vi "GetTargetCandidates.vi"(9 "Minimum Area":dbl, 10 "HSL Range":T3={"Hue"={0.0, 6.122448979591837}, "Saturation"={0.0, 6.122448979591837}, "Luminance"={0.0, 6.122448979591837}} {"Luminance" scale=0.0..255.0; "Saturation" scale=0.0..255.0; "Hue" scale=0.0..255.0}, 11 "Image":T2) -> (1 "Thresholded Image":T2, 2 "Horizontal Targets":T1[](array[typedef]), 3 "Vertical Targetss":T1[](array[typedef]))   [LabVIEW 2013]
uses:
  <vilib>/vision/Image Controls.llb/IMAQ Image.ctl
  HSLRange.ctl
  Target Type.ctl
  <vilib>/vision/NI_Vision_Development_Module.lvlib
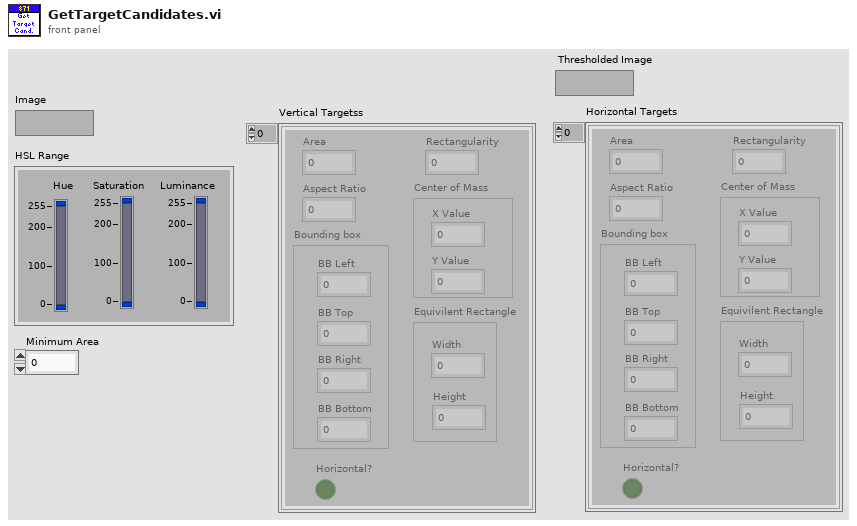
[diagram p1: front panel]
types:
  T1 = typedef "Target Type.ctl" = cluster{"Area":dbl, "Bounding box":cluster{"BB Left":dbl, "BB Top":dbl, "BB Right":dbl, "BB Bottom":dbl}, "Center of Mass":cluster{"X Value":dbl, "Y Value":dbl}, "Equivilent Rectangle":cluster{"Width":dbl, "Height":dbl}, "Aspect Ratio":dbl, "Rectangularity":dbl, "Horizontal?":bool}
  T2 = typedef "IMAQ Image.ctl" = refnum<image>
  T3 = typedef "HSLRange.ctl" = cluster{"Hue":cluster{dbl, dbl}, "Saturation":cluster{dbl, dbl}, "Luminance":cluster{dbl, dbl}}
  T4 = typedef "Particle Parameters" = i32
  T5 = typedef "Image Type" = u32
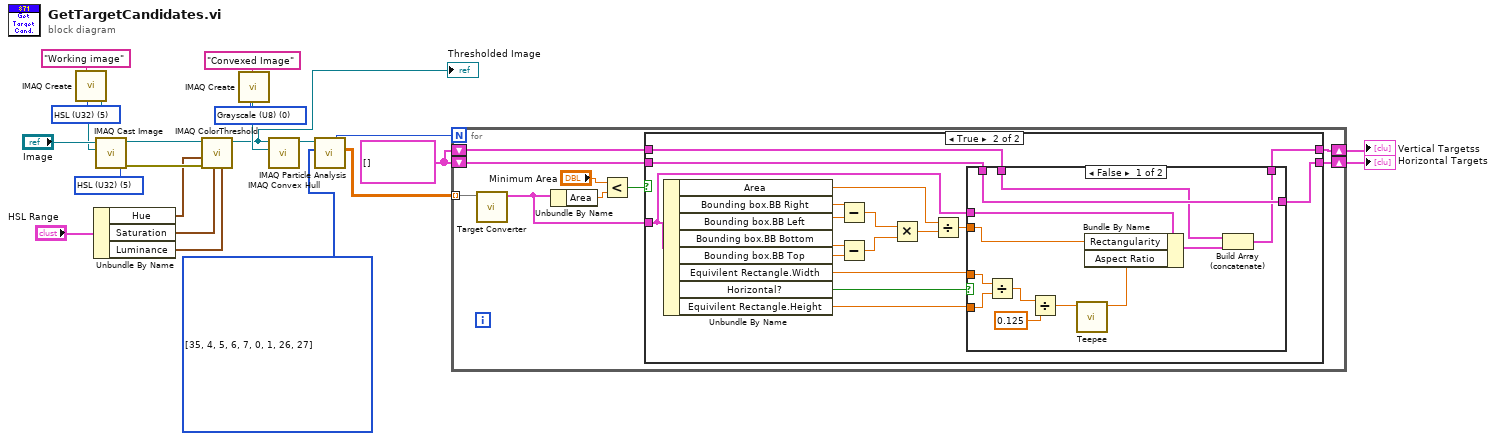
[diagram p0: block diagram]
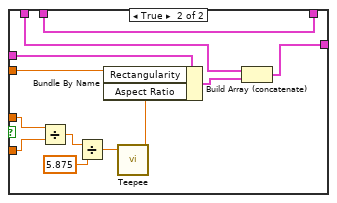
[diagram p3: hidden frame]
diagram:
  w4 = T4[] [35, 4, 5, 6, 7, 0, 1, 26, 27] items=["Center of Mass X", "Center of Mass Y", "First Pixel X", "First Pixel Y", "Bounding Rect Left", "Bounding Rect Top", "Bounding Rect Right", "Bounding Rect Bottom", "Max Feret Diameter Start X", "Max Feret Diameter Start Y", "Max Feret Diameter End X", "Max Feret Diameter End Y", "Max Horiz. Segment Length Left", "Max Horiz. Segment Length Right", "Max Horiz. Segment Length Row", "-", "Bounding Rect Width", "Bounding Rect Height", "Bounding Rect Diagonal", "Perimeter", "Convex Hull Perimeter", "Holes' Perimeter", "Max Feret Diameter", "Equivalent Ellipse Major Axis", "Equivalent Ellipse Minor Axis", "Equivalent Ellipse Minor Axis (Feret)", "Equivalent Rect Long Side", "Equivalent Rect Short Side", "Equivalent Rect Diagonal", "Equivalent Rect Short Side (Feret)", "Average Horiz. Segment Length", "Average Vert. Segment Length", "Hydraulic Radius", "Waddel Disk Diameter", "-", "Area", "Holes' Area", "Particle & Holes' Area", "Convex Hull Area", "Image Area", "-", "Number of Holes", "Number of Horiz. Segments", "Number of Vert. Segments", "-", "Orientation", "Max Feret Diameter Orientation", "-", "% Area/Image Area", "% Area/(Particle & Holes' Area)", "Ratio of Equivalent Ellipse Axes", "Ratio of Equivalent Rect Sides", "-", "Elongation Factor", "Compactness Factor", "Heywood Circularity Factor", "Type Factor", "-", "Sum X", "Sum Y", "Sum XX", "Sum XY", "Sum YY", "Sum XXX", "Sum XXY", "Sum XYY", "Sum YYY", "-", "Moment of Inertia XX", "Moment of Inertia XY", "Moment of Inertia YY", "Moment of Inertia XXX", "Moment of Inertia XXY", "Moment of Inertia XYY", "Moment of Inertia YYY", "Norm. Moment of Inertia XX", "Norm. Moment of Inertia XY", "Norm. Moment of Inertia YY", "Norm. Moment of Inertia XXX", "Norm. Moment of Inertia XXY", "Norm. Moment of Inertia XYY", "Norm. Moment of Inertia YYY", "Hu Moment 1", "Hu Moment 2", "Hu Moment 3", "Hu Moment 4", "Hu Moment 5", "Hu Moment 6", "Hu Moment 7"] ("Pixel Measurements")
  w3 = T1[] []
  w11 = T5 0 items=["Grayscale (U8)", "Grayscale (I16)", "Grayscale (SGL)", "Complex (CSG)", "RGB (U32)", "HSL (U32)", "RGB (U64)", "Grayscale (U16)"] ("Image Type")
  w18 = T5 5 items=["Grayscale (U8)", "Grayscale (I16)", "Grayscale (SGL)", "Complex (CSG)", "RGB (U32)", "HSL (U32)", "RGB (U64)", "Grayscale (U16)"] ("Image Type")
  w22 = T5 5 items=["Grayscale (U8)", "Grayscale (I16)", "Grayscale (SGL)", "Complex (CSG)", "RGB (U32)", "HSL (U32)", "RGB (U64)", "Grayscale (U16)"] ("Image Type")
  n1 = call "IMAQ Create"("Image Name"="Working image", "Image Type"=w18) -> ("New Image"=w16:T2)  [unwired: 3 in, 1 out]
  n2 = Unbundle By Name("HSL Range") -> ("Hue"=w14:cluster{dbl, dbl}, "Saturation"=w13:cluster{dbl, dbl}, "Luminance"=w12:cluster{dbl, dbl})
  n3 = call "IMAQ Cast Image"("Image Type"=w22, "Image Dst"=w16, "Image Src"="Image") -> ("error out"=w17:errorcluster, "Image Dst Out"=w20:T2)  [unwired: 7 in]
  n4 = call "IMAQ ColorThreshold"("Blue or Luma or Val or Inten Range"=w12, "Green or Sat Range"=w13, "error in (no error)"=w17, "Red or Hue Range"=w14, "Image Src"=w20) -> ("Image Dst Out"=w5:T2)  [unwired: 5 in, 1 out]
  "Thresholded Image" <- w5
  n5 = call "IMAQ Create"("Image Name"="Convexed Image", "Image Type"=w11) -> ("New Image"=w9:T2)  [unwired: 3 in, 1 out]
  n6 = call "IMAQ Convex Hull"("Image Dst"=w9, "Image Src"=w5) -> ("Image Dst Out"=w8:T2)  [unwired: 8 in, 1 out]
  n7 = call "IMAQ Particle Analysis"("Pixel Measurements"=w4, "Image"=w8) -> ("Particle Measurements (Pixels)"=w6:dbl[][], "Number of Particles"=w7:i32)  [unwired: 4 in, 4 out]
  n8 = for {
    N: w7 -> [_]
    shift-right: [w28] -> w2
    shift-left: w3 -> [w27]
    tunnel: w6 -> [w26] mode=indexing
    shift-right: [w23] -> w1
    shift-left: w3 -> [w24]
    n9 = call "Target Converter.vi"("Array"=w26) -> ("Target type"=w25:T1)  [unwired: 10 in]
    n10 = Unbundle By Name(w25) -> ("Area"=w30:dbl)
    n11 = Less?(x="Minimum Area", y=w30) -> (x < y?=w29:bool)
    n12 = case shown="True" w29 {
      tunnel: [w33 w42] -> w28
      tunnel: w27 -> [w33 w34]
      tunnel: w25 -> [_ w38]
      tunnel: w24 -> [w32 w35]
      tunnel: [w32 w36] -> w23
      frame False {
      }
      frame True {
        n13 = Unbundle By Name(w38) -> ("Area"=w45:dbl, "Bounding box.BB Right"=w50:dbl, "Bounding box.BB Left"=w49:dbl, "Bounding box.BB Bottom"=w48:dbl, "Bounding box.BB Top"=w47:dbl, "Equivilent Rectangle.Width"=w40:dbl, "Horizontal?"=w41:bool, "Equivilent Rectangle.Height"=w39:dbl)
        n14 = Subtract(x=w50, y=w49) -> (x-y=w44:dbl)
        n15 = Subtract(x=w48, y=w47) -> (x-y=w43:dbl)
        n16 = Multiply(x=w44, y=w43) -> (x*y=w46:dbl)
        n17 = Divide(x=w45, y=w46) -> (x/y=w37:dbl)
        n18 = case shown="False" w41 {
          tunnel: w40 -> [w62 w74]
          tunnel: w39 -> [w61 w73]
          tunnel: [w51 w63] -> w42
          tunnel: w38 -> [w54 w69]
          tunnel: w37 -> [w52 w67]
          tunnel: [w57 w65] -> w36
          tunnel: w35 -> [w57 w64]
          tunnel: w34 -> [w53 w63]
          frame False {
            n19 = Divide(x=w62, y=w61) -> (x/y=w59:dbl)
            n20 = Divide(x=w59, y=0.125) -> (x/y=w58:dbl)
            n21 = call "Teepee.vi"("Actual"=w58) -> ("Teepee-ed"=w55:dbl)  [unwired: 10 in]
            n22 = Bundle By Name(cluster=w54, "Rectangularity"=w52, "Aspect Ratio"=w55) -> (w56:T1)
            n23 = Build Array (concatenate)(w53, w56) -> (w51:T1[])
          }
          frame True {
            n24 = Divide(x=w74, y=w73) -> (x/y=w71:dbl)
            n25 = Divide(x=w71, y=5.875) -> (x/y=w70:dbl)
            n26 = call "Teepee.vi"("Actual"=w70) -> ("Teepee-ed"=w68:dbl)  [unwired: 10 in]
            n27 = Bundle By Name(cluster=w69, "Rectangularity"=w67, "Aspect Ratio"=w68) -> (w66:T1)
            n28 = Build Array (concatenate)(w64, w66) -> (w65:T1[])
          }
        }
      }
    }
  }
  "Vertical Targetss" <- w2
  "Horizontal Targets" <- w1
